vi "copy Complex Data to Array 2D.vi"(4 "error in (no error)":errorcluster, 7 "Complex Data":refnum<class "Complex Data.lvclass">) -> (0 "error out":errorcluster, 2 "Data Content":csg[][](array[numeric]), 3 "Complex Data out":refnum<class "Complex Data.lvclass">)   [LabVIEW 2018]
doc: "Copies the real and imaginary parts of the Complex Data object to 2D array of Float32."
uses:
  SpectralRadar/LabVIEW/2012/user.lib/SpectralRadar.llb/Complex Data.lvclass
  SpectralRadar/LabVIEW/2012/user.lib/SpectralRadar.llb/Data Property Int Selection.ctl
  SpectralRadar/LabVIEW/2012/user.lib/SpectralRadar.llb/Data.lvclass
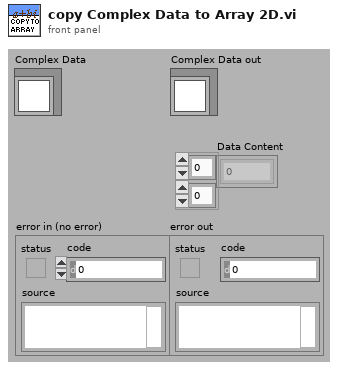
[diagram p1: front panel]
types:
  T1 = typedef "Data.lvclass/Data Property Int Selection.ctl" = enum16{"Dimensions", "Size 1", "Size 2", "Size 3", "Number of Data Points", "Data Size in Bytes", "Bytes per Pixel"}
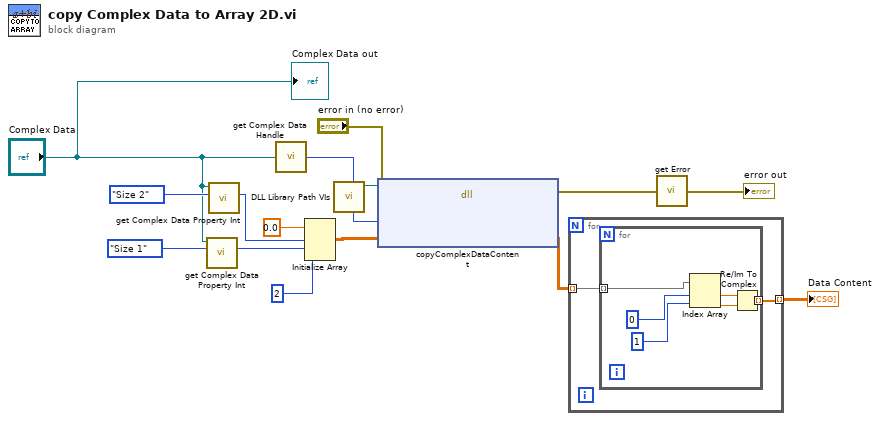
[diagram p0: block diagram]
diagram:
  n1 = call "get Complex Data Property Int.vi"("Data Property Selection"=Data_Property_Int_Selection."Size 1", "Complex Data"="Complex Data") -> ("Property Value"=w3:i32)  [unwired: 3 in, 2 out]
  n2 = call "get Complex Data Property Int.vi"("Data Property Selection"=Data_Property_Int_Selection."Size 2", "Complex Data"="Complex Data") -> ("Property Value"=w4:i32)  [unwired: 3 in, 2 out]
  n3 = call "get Complex Data Handle.vi"("Complex Data"="Complex Data") -> ("Handle"=w5:u64)
  n4 = Initialize Array(sgl 0.0 ("element"), w4, w3, 2 ("dimension size")) -> (w9:sgl[][][])
  n5 = call "DLL Library Path VIs.vi"() -> ("SpectralRadarDLL"=w1:path)  [unwired: 8 in, 3 out]
  n6 = dll-call lib="C:/Project/SerialSectOCT - FFT GPU/SerialSectOCT/Labview Software/DLL/SpectralRadar.dll" fn="copyComplexDataContent"(path in=w1, error in="error in (no error)", "Data Handle"=w5, "Data Content"=w9) -> (error out=w13:errorcluster, "Data Content"=w8:sgl[][][])  [unwired: 3 in, 1 out]
  n7 = for {
    tunnel: w8 -> [w17] mode=indexing
    tunnel: [w16] -> w7 mode=indexing
    n8 = for {
      tunnel: w17 -> [w23] mode=indexing
      tunnel: [w18] -> w16 mode=indexing
      n9 = Index Array(array=w23, index #1=0 ("index"), index #2=1 ("index")) -> (element #1=w20:sgl, element #2=w19:sgl)
      n10 = Re/Im To Complex(1:w19, 2:w20) -> (0:w18:csg)
    }
  }
  "Data Content" <- w7
  n11 = call "get Error.vi"("error in (no error)"=w13) -> ("error out"=→"error out":errorcluster)
  "Complex Data out" <- "Complex Data"
